vi "Correct Tau for Rayleigh.vi"(8 "error in (no error)":errorcluster, 11 "CRDS Cell in":refnum<class "CRDS Cell.lvclass">) -> (0 "error out":errorcluster, 3 "CRDS Cell Out":refnum<class "CRDS Cell.lvclass">)   [LabVIEW 2019, in "CRDS Cell.lvclass"]
uses:
  CRDS Cell.lvclass
  CRDS Cell.lvclass/CRDS Cell.ctl
  Data/Cell/CRDS Cell Data.lvclass/CRDS Cell Data.ctl
  Data/Cell/Read extParam.vi
  Data/Cell/Write extParam.vi
  Data/Cell/Read hkParam.vi
  General/Atmospheric/Atmospheric Constants.vi
  General/Atmospheric/Atmospheric Library.lvlib
  Data/Cell/CRDS Cell Data.lvclass
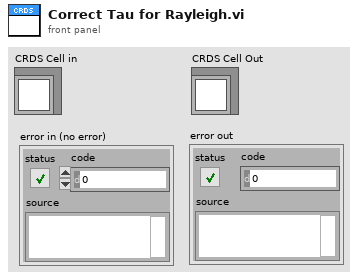
[diagram p1: front panel]
types:
  T1 = typedef "Base CRDS Lib.lvlib/calData.ctl" = cluster{"rhDilFac":sgl, "Q":sgl, "Tmean":sgl, "extDilFac":sgl, "rhCell":sgl, "P":sgl, "T":sgl}
  T2 = typedef "extparam.ctl" = cluster{"Tau":sgl, "Tau0cor":sgl, "ext":sgl, "extCorr":sgl, "stdevTau":sgl, "eTau":sgl, "taucorr":sgl, "Tau0":sgl, "max":sgl}
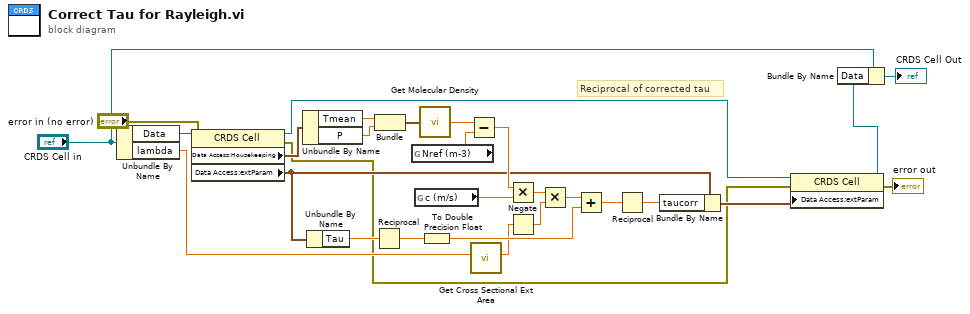
[diagram p0: block diagram]
diagram:
  # "Reciprocal of corrected tau"
  n1 = Unbundle By Name("CRDS Cell in") -> ("Data"=w14:refnum<class "CRDS Cell Data.lvclass">, "lambda"=w12:dbl)
  n2 = property class="CRDS Cell"(reference=w14, error in="error in (no error)") -> (reference out=w9:refnum<class "CRDS Cell Data.lvclass">, error out=w2:errorcluster, "Data Access:Housekeeping"=w13:T1, "Data Access:extParam"=w8:T2)
  n3 = Unbundle By Name(w13) -> ("Tmean"=w15:sgl, "P"=w16:sgl)
  n4 = Unbundle By Name(w8) -> ("Tau"=w11:sgl)
  n5 = Reciprocal(x=w11) -> (1/x=w19:sgl)
  n6 = Bundle("Tmean"=w15, "P"=w16) -> (w24:cluster{"Tmean":sgl, "P":sgl})  [unwired: 1 in]
  n7 = global read "Atmospheric Constants.vi" "Nref (m-3)"() -> (w17:dbl)
  n8 = global read "Atmospheric Constants.vi" "c (m/s)"() -> (w21:dbl)
  n9 = call "Get Molecular Density.vi"("thermoCond"=w24) -> ("M (m-3)"=w23:dbl)
  n10 = To Double Precision Float(number=w19) -> (double precision float=w28:dbl)
  n11 = Subtract(x=w23, y=w17) -> (x-y=w20:dbl)
  n12 = call "Get Cross Sectional Ext Area.vi"("l (nm)"=w12) -> ("CAext (m2)"=w25:dbl)  [unwired: 10 in]
  n13 = Multiply(x=w20, y=w21) -> (x*y=w18:dbl)
  n14 = Negate(x=w25) -> (-x=w26:dbl)
  n15 = Multiply(x=w18, y=w26) -> (x*y=w27:dbl)
  n16 = Add(x=w27, y=w28) -> (x+y=w22:dbl)
  n17 = Reciprocal(x=w22) -> (1/x=w6:dbl)
  n18 = Bundle By Name(cluster=w8, "taucorr"=w6) -> (w7:T2)
  n19 = property class="CRDS Cell"(reference=w9, error in=w2, "Data Access:extParam"=w7) -> (reference out=w5:refnum<class "CRDS Cell Data.lvclass">, error out=→"error out":errorcluster)
  n20 = Bundle By Name(cluster="CRDS Cell in", "Data"=w5) -> (→"CRDS Cell Out":refnum<class "CRDS Cell.lvclass">)
